vi "Get Name.vi"(8 "error in (no error)":errorcluster, 11 "Blueprint in":refnum<class "Blueprint.lvclass">) -> (0 "error out":errorcluster, 2 "Name":string, 3 "Blueprint out":refnum<class "Blueprint.lvclass">)   [LabVIEW 2020, in "Blueprint.lvclass"]
uses:
  Blueprint.lvclass
  Blueprint.lvclass/Blueprint.ctl
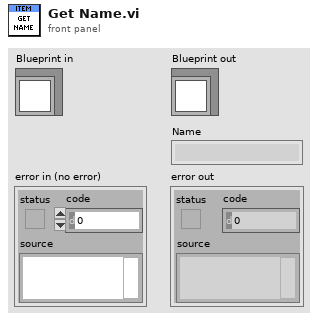
[diagram p1: front panel]
types:
  T1 = typedef "Blueprint.lvclass/Ref Data.ctl" = cluster{"Ingredients":T2[], "Workstation":refnum<class "Workstation.lvclass">, "Craft Time":dbl, "Name":string}
  T2 = typedef "Item.lvclass/Ingredient.ctl" = cluster{"Item":refnum<class "Item.lvclass">, "Qty":dbl}
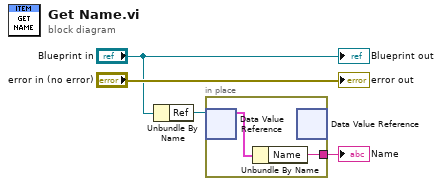
[diagram p0: block diagram]
diagram:
  n1 = Unbundle By Name("Blueprint in") -> ("Ref"=w3:refnum<data-value>)
  n2 = in-place {
    in-place-border: [w5] -> w1
    n3 = in-place-dvr #1(w3) -> (w6:T1)  [unwired: 1 out]
    n4 = Unbundle By Name(w6) -> ("Name"=w5:string)
    n5 = in-place-dvr #1() -> ()  [unwired: 1 in, 2 out]
  }
  "Name" <- w1
  "error out" <- "error in (no error)"
  "Blueprint out" <- "Blueprint in"
